vi "CorrelImages (SubVI).vi"(8 "last drift detected":i32, 9 "Correlate":u16(ring) items=["first Frame", "successive Frames"], 10 "Ref Array":dbl[][][](array[numeric]), 11 "New Image":dbl[][](array[numeric])) -> (2 "Y drift":i32, 3 "X drift":i32, 4 "Ref Array out":dbl[][][](array[numeric]), 5 "Queue Steps":i32=40)   [LabVIEW 2014]
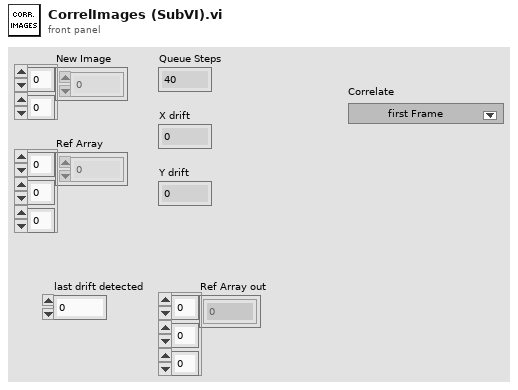
[diagram p1: front panel]
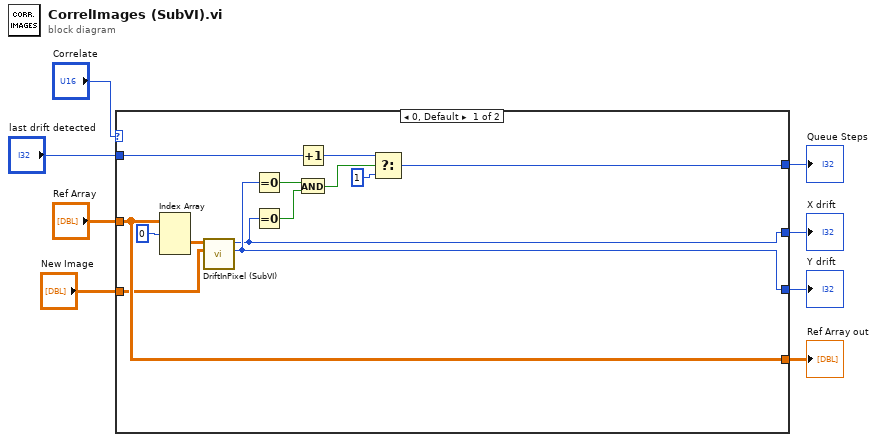
[diagram p0: block diagram]
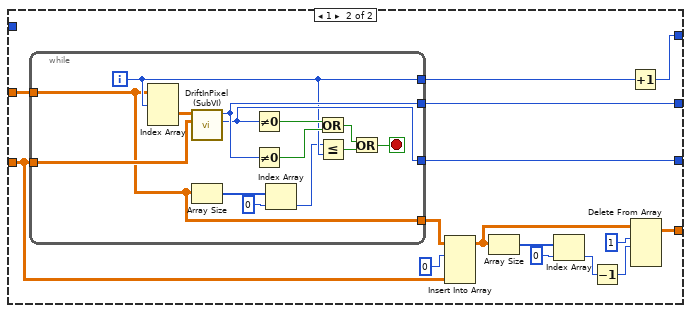
[diagram p2: hidden frame]
diagram:
  n1 = case shown="0, Default" "Correlate" {
    tunnel: [w12 w22] -> w8
    tunnel: [w17 w35] -> w7
    tunnel: [w16 w34] -> w6
    tunnel: [w20 w27] -> w5
    tunnel: "New Image" -> [w18 w25]
    tunnel: "Ref Array" -> [w20 w23]
    tunnel: "last drift detected" -> [w10 _]
    frame 0, Default {
      n2 = Index Array(array=w20, index (dim 0)=0 ("index (page)")) -> (element=w19:dbl[][])  [unwired: 2 in]
      n3 = call "DriftInPixel (SubVI).vi"("New image"=w18, "Ref image"=w19) -> ("Y drift"=w17:i32, "X drift"=w16:i32)  [unwired: 7 in, 1 out]
      n4 = Equal To 0?(x=w17) -> (x = 0?=w15:bool)
      n5 = Equal To 0?(x=w16) -> (x = 0?=w14:bool)
      n6 = Increment(x=w10) -> (x+1=w9:i32)
      n7 = And(x=w15, y=w14) -> (x .and. y?=w13:bool)
      n8 = Select(t=w9, s=w13, f=1) -> (s? t:f=w12:i32)
    }
    frame 1 {
      n9 = while {
        tunnel: w25 -> [w48]
        tunnel: w23 -> [w38]
        tunnel: [w47] -> w34
        tunnel: [w46] -> w35
        tunnel: [w42] -> w36
        tunnel: [w38] -> w24
        i -> [w42]
        stop <- w44 stop-if-true
        n10 = Index Array(array=w38, index (dim 0)=w42) -> (element=w37:dbl[][])  [unwired: 2 in]
        n11 = call "DriftInPixel (SubVI).vi"("New image"=w48, "Ref image"=w37) -> ("Y drift"=w46:i32, "X drift"=w47:i32)  [unwired: 7 in, 1 out]
        n12 = Array Size(array=w38) -> (size(s)=w41:i32[])
        n13 = Not Equal To 0?(x=w46) -> (x != 0?=w50:bool)
        n14 = Not Equal To 0?(x=w47) -> (x != 0?=w49:bool)
        n15 = Index Array(array=w41, index=0) -> (element=w39:i32)
        n16 = Or(x=w50, y=w49) -> (x .or. y?=w45:bool)
        n17 = Less Or Equal?(x=w39, y=w42) -> (x <= y?=w43:bool)
        n18 = Or(x=w45, y=w43) -> (x .or. y?=w44:bool)
      }
      n19 = Insert Into Array(array=w24, index (dim 0)=0 ("index (page)"), new element=w25) -> (w28:dbl[][][])  [unwired: 2 in]
      n20 = Array Size(array=w28) -> (size(s)=w29:i32[])
      n21 = Index Array(array=w29, index=0) -> (element=w31:i32)
      n22 = Decrement(x=w31) -> (x-1=w32:i32)
      n23 = Increment(x=w36) -> (x+1=w22:i32)
      n24 = Delete From Array(array=w28, length=1, index (dim 0)=w32) -> (array with subset deleted=w27:dbl[][][])  [unwired: 2 in, 1 out]
    }
  }
  "Queue Steps" <- w8
  "Y drift" <- w7
  "X drift" <- w6
  "Ref Array out" <- w5
